vi "DDC Stage 01 - 1Ch.vi"(0 "data in":T1[](array[typedef])=[{"I"=0.0, "Q"=0.0, "overflow"=FALSE}, {"I"=0.0, "Q"=0.0, "overflow"=FALSE}, {"I"=0.0, "Q"=0.0, "overflow"=FALSE}, {"I"=0.0, "Q"=0.0, "overflow"=FALSE}, {"I"=0.0, "Q"=0.0, "overflow"=FALSE}, {"I"=0.0, "Q"=0.0, "overflow"=FALSE}, {"I"=0.0, "Q"=0.0, "overflow"=FALSE}, {"I"=0.0, "Q"=0.0, "overflow"=FALSE}], 1 "acq.reset":bool, 9 "input valid":bool, 12 "ddc.freq.shift":fxp<+/-,48,0>[](array[numeric])=[0.0, 0.0, 0.0, 0.0, 0.0, 0.0, 0.0, 0.0, 0.0, 0.0, 0.0, 0.0, 0.0, 0.0, 0.0, 0.0] format="%.48g", 13 "ddc.phase":fxp<+/-,21,0>[](array[numeric])=[0.0, 0.0, 0.0, 0.0, 0.0, 0.0, 0.0, 0.0, 0.0, 0.0, 0.0, 0.0, 0.0, 0.0, 0.0, 0.0] format="%.21g") -> (3 "CHs overflow":bool, 10 "FIFOs Timeout":bool)   [LabVIEW 2015, in "DDC_7976R_v1.lvlib"]
uses:
  DDC_7976R_v1.lvlib
  <instrlib>/_niInstr/DSP/v1/Shared/Public/IQ Data.ctl
  Private/Typedef - internal -01.ctl
  <instrlib>/_niInstr/DSP/v1/Shared/niInstr DSP v1 Shared.lvlib
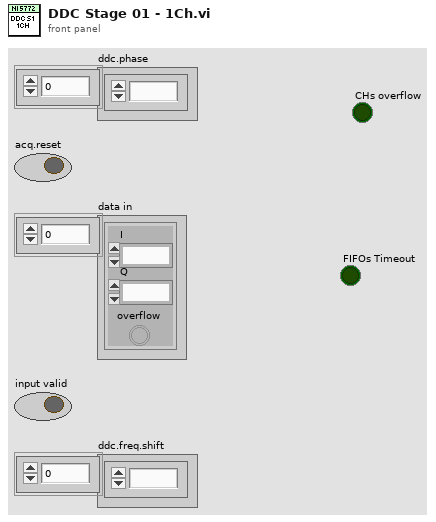
[diagram p1: front panel]
types:
  T1 = typedef "niInstr DSP v1 Shared.lvlib/IQ Data.ctl" = cluster{"I":fxp<+/-,18,1>, "Q":fxp<+/-,18,1>, "overflow":bool}
  T2 = typedef "DDC_7976R_v1.lvlib/Typedef - internal -01.ctl" = cluster{"acq.reset":bool, "data in":T1[], "input valid":bool, "ddc.freq.shift":fxp<+/-,48,0>[], "ddc.phase":fxp<+/-,21,0>[]}
  T3 = typedef "DDC_7976R_v1.lvlib/Typedef - internal -02.ctl" = cluster{"DSP Overflow":bool, "Timed Out?":bool}
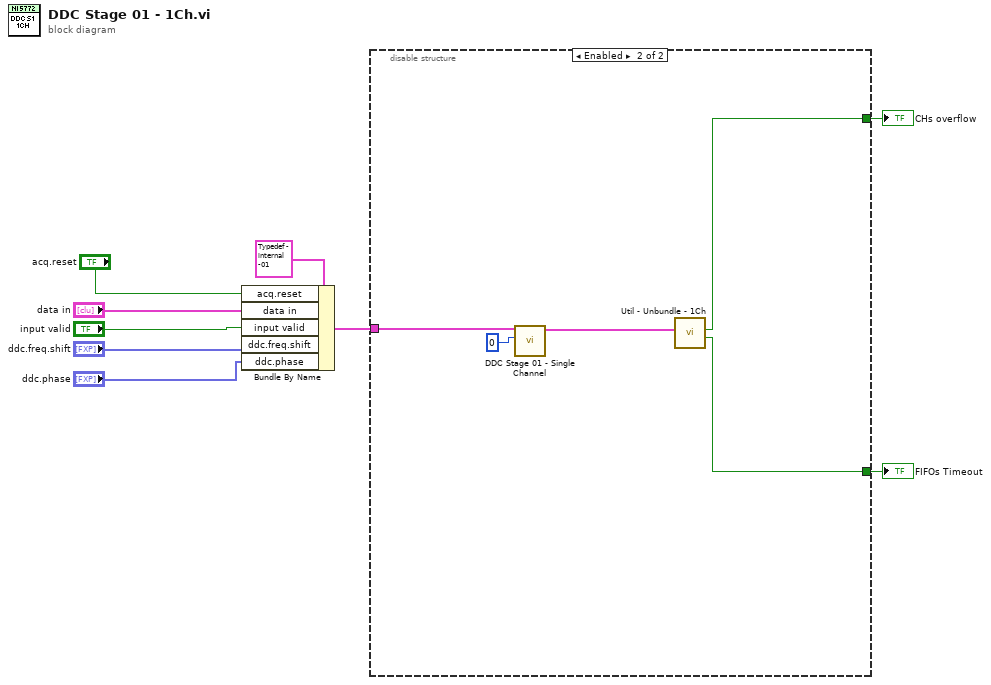
[diagram p0: block diagram]
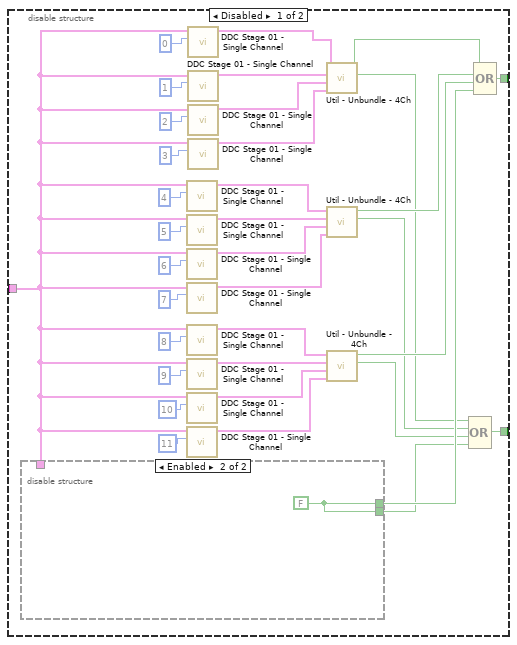
[diagram p2: hidden frame]
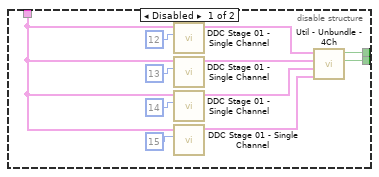
[diagram p3: hidden frame]
diagram:
  n1 = Bundle By Name(cluster=T2 {"acq.reset"=FALSE, "data in"=[{"I"=0.0, "Q"=0.0, "overflow"=FALSE}, {"I"=0.0, "Q"=0.0, "overflow"=FALSE}, {"I"=0.0, "Q"=0.0, "overflow"=FALSE}, {"I"=0.0, "Q"=0.0, "overflow"=FALSE}, {"I"=0.0, "Q"=0.0, "overflow"=FALSE}, {"I"=0.0, "Q"=0.0, "overflow"=FALSE}, {"I"=0.0, "Q"=0.0, "overflow"=FALSE}, {"I"=0.0, "Q"=0.0, "overflow"=FALSE}], "input valid"=FALSE, "ddc.freq.shift"=[0.0, 0.0, 0.0, 0.0, 0.0, 0.0, 0.0, 0.0, 0.0, 0.0, 0.0, 0.0, 0.0, 0.0, 0.0, 0.0], "ddc.phase"=[0.0, 0.0, 0.0, 0.0, 0.0, 0.0, 0.0, 0.0, 0.0, 0.0, 0.0, 0.0, 0.0, 0.0, 0.0, 0.0]} ("output cluster"), "acq.reset"="acq.reset", "data in"="data in", "input valid"="input valid", "ddc.freq.shift"="ddc.freq.shift", "ddc.phase"="ddc.phase") -> (w3:T2)
  n2 = disable-structure shown="Enabled" {
    disable-tunnel: w3 -> [w30 w60]
    disable-tunnel: [w11 w57] -> w2
    disable-tunnel: [w10 w58] -> w1
    frame Disabled {
      n3 = disable-structure shown="Enabled" {
        disable-tunnel: w30 -> [w51 _]
        disable-tunnel: [w46 w56] -> w16
        disable-tunnel: [w45 w56] -> w12
        frame Disabled {
          n4 = call "DDC Stage 01 - Single Channel.vi"("ch #"=12, "input cluster"=w51) -> ("output"=w49:T3)  [unwired: 9 in]
          n5 = call "DDC Stage 01 - Single Channel.vi"("ch #"=13, "input cluster"=w51) -> ("output"=w50:T3)  [unwired: 9 in]
          n6 = call "DDC Stage 01 - Single Channel.vi"("ch #"=14, "input cluster"=w51) -> ("output"=w48:T3)  [unwired: 9 in]
          n7 = call "DDC Stage 01 - Single Channel.vi"("ch #"=15, "input cluster"=w51) -> ("output"=w47:T3)  [unwired: 9 in]
          n8 = call "Util - Unbundle - 4Ch.vi"("in3"=w47, "in2"=w48, "in1"=w50, "in0"=w49) -> ("Timed Out?"=w45:bool, "DSP Overflow"=w46:bool)  [unwired: 6 in]
        }
        frame Enabled {
          w56 = FALSE ("DSP Overflow")
        }
      }
      n9 = call "DDC Stage 01 - Single Channel.vi"("ch #"=4, "input cluster"=w30) -> ("output"=w25:T3)  [unwired: 9 in]
      n10 = call "DDC Stage 01 - Single Channel.vi"("ch #"=5, "input cluster"=w30) -> ("output"=w27:T3)  [unwired: 9 in]
      n11 = call "DDC Stage 01 - Single Channel.vi"("ch #"=6, "input cluster"=w30) -> ("output"=w24:T3)  [unwired: 9 in]
      n12 = call "DDC Stage 01 - Single Channel.vi"("ch #"=7, "input cluster"=w30) -> ("output"=w23:T3)  [unwired: 9 in]
      n13 = call "DDC Stage 01 - Single Channel.vi"("ch #"=8, "input cluster"=w30) -> ("output"=w22:T3)  [unwired: 9 in]
      n14 = call "DDC Stage 01 - Single Channel.vi"("ch #"=9, "input cluster"=w30) -> ("output"=w26:T3)  [unwired: 9 in]
      n15 = call "DDC Stage 01 - Single Channel.vi"("ch #"=10, "input cluster"=w30) -> ("output"=w21:T3)  [unwired: 9 in]
      n16 = call "DDC Stage 01 - Single Channel.vi"("ch #"=11, "input cluster"=w30) -> ("output"=w20:T3)  [unwired: 9 in]
      n17 = call "DDC Stage 01 - Single Channel.vi"("ch #"=0, "input cluster"=w30) -> ("output"=w43:T3)  [unwired: 9 in]
      n18 = call "DDC Stage 01 - Single Channel.vi"("ch #"=1, "input cluster"=w30) -> ("output"=w41:T3)  [unwired: 9 in]
      n19 = call "DDC Stage 01 - Single Channel.vi"("ch #"=2, "input cluster"=w30) -> ("output"=w29:T3)  [unwired: 9 in]
      n20 = call "DDC Stage 01 - Single Channel.vi"("ch #"=3, "input cluster"=w30) -> ("output"=w28:T3)  [unwired: 9 in]
      n21 = call "Util - Unbundle - 4Ch.vi"("in3"=w28, "in2"=w29, "in1"=w41, "in0"=w43) -> ("Timed Out?"=w15:bool, "DSP Overflow"=w19:bool)  [unwired: 6 in]
      n22 = call "Util - Unbundle - 4Ch.vi"("in3"=w23, "in2"=w24, "in1"=w27, "in0"=w25) -> ("Timed Out?"=w14:bool, "DSP Overflow"=w18:bool)  [unwired: 6 in]
      n23 = call "Util - Unbundle - 4Ch.vi"("in3"=w20, "in2"=w21, "in1"=w26, "in0"=w22) -> ("Timed Out?"=w13:bool, "DSP Overflow"=w17:bool)  [unwired: 6 in]
      n24 = Compound Arithmetic op=OR(w15, w14, w13, w12) -> (w10:bool)
      n25 = Compound Arithmetic op=OR(w19, w18, w17, w16) -> (w11:bool)
    }
    frame Enabled {
      n26 = call "DDC Stage 01 - Single Channel.vi"("ch #"=0, "input cluster"=w60) -> ("output"=w59:T3)  [unwired: 9 in]
      n27 = call "Util - Unbundle - 1Ch.vi"("output"=w59) -> ("Timed Out?"=w58:bool, "DSP Overflow"=w57:bool)  [unwired: 9 in]
    }
  }
  "CHs overflow" <- w2
  "FIFOs Timeout" <- w1
